vi "Spuler_interactive_lock_routine.vi"() -> ()   [LabVIEW 2012]
uses:
  <vilib>/DAQmx/write.llb/DAQmx Write (Digital 1D Bool NChan 1Samp 1Line).vi
  <vilib>/DAQmx/miscellaneous.llb/DAQmx Fill In Error Info.vi
  H2O_DIAL/LabVIEW-2012/Bristol WM V2_31b/CLDevIFace.dll
panel:
  out "On Diff read (nm)":dbl=2.73590208053065e-05 format="%_7g"
  in  "Lambda On Set (nm)":dbl=828.195 format="%#.5f"
  out "Online Lock":bool=TRUE
  out "Lambda On Read (nm)":dbl=828.1950273590209 format="%.5f"
  in  "Bristol In":i32=5
  in  "exit":bool
  out "WM Switch":bool=TRUE
  in  "WL Diff Allowed (nm)":dbl=5e-05 format="%#_15g"
  out "Off Diff read (nm)":dbl=2.4793750640128565e-05 format="%_7g"
  in  "Lambda Off Set (nm)":dbl=828.29425 format="%#.5f"
  out "Ofline Lock":bool=TRUE
  out "Lambda Off Read (nm)":dbl=828.2942747937507 format="%.5f"
  in  "Settings":T1={"Module"=enum."Etalon TEC", "OnLineTEC"=19.599694999999315, "OnLineLD"=0.15, "OffLineTEC"=17.258364999999106, "OffLineLD"=0.155, "EtalonTEC"=26.25, "TSOA-TEC"=18.0} {"OffLineLD" min=0.0 max=0.175 step=0.001 format="%.3p"; "OnLineLD" min=0.0 max=0.175 step=0.001 format="%.3p"; "TSOA-TEC" format="%.2g"; "EtalonTEC" format="%.2g"; "OffLineTEC" min=0.0 max=30.0 step=0.1 format="%.3g"; "OnLineTEC" min=0.0 max=30.0 step=0.1 format="%.3g"}
  out "Readings":T2={"OnLineTEC"=19.5938969, "OnLineLD"=0.150162116, "OffLineTEC"=17.2649479, "OffLineLD"=0.154738292, "EtalonTEC"=26.2012253, "TSOA-TEC"=18.0232182, "Pro8000"=TRUE, "OnLine TEC"=TRUE, "OnLine LD"=TRUE, "OffLine TEC"=TRUE, "OffLine LD"=TRUE, "Etalon TEC"=TRUE, "TSOA TEC"=TRUE} {"OffLineLD" format="%.4g"; "OnLineLD" format="%.4g"; "TSOA-TEC" format="%.3g"; "EtalonTEC" format="%.3g"; "OffLineTEC" format="%.3g"; "OnLineTEC" format="%.3g"}
  out "Bristol Out":i32=13
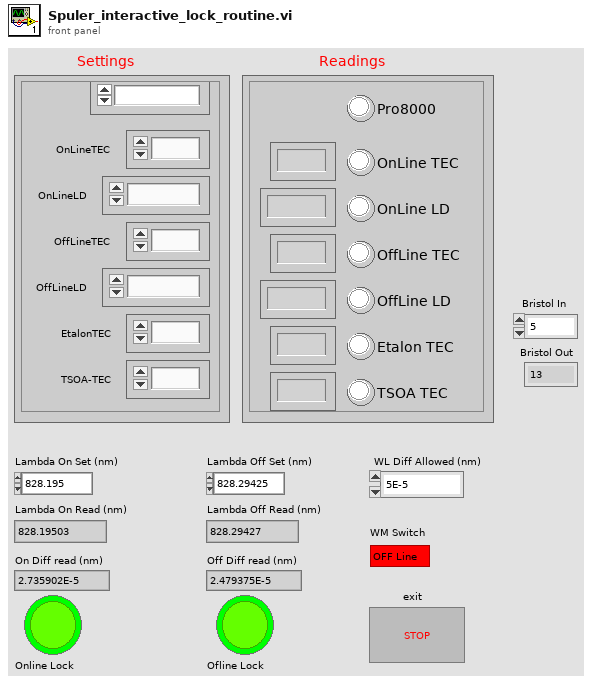
[diagram p1: front panel]
types:
  T1 = cluster{"Module":enum16{"On Line TEC", "On Line LD", "Off Line TEC", "Off Line LD", "Etalon TEC", "TSOA TEC"}, "OnLineTEC":dbl, "OnLineLD":dbl, "OffLineTEC":dbl, "OffLineLD":dbl, "EtalonTEC":dbl, "TSOA-TEC":dbl}
  T2 = cluster{"OnLineTEC":dbl, "OnLineLD":dbl, "OffLineTEC":dbl, "OffLineLD":dbl, "EtalonTEC":dbl, "TSOA-TEC":dbl, "Pro8000":bool, "OnLine TEC":bool, "OnLine LD":bool, "OffLine TEC":bool, "OffLine LD":bool, "Etalon TEC":bool, "TSOA TEC":bool}
  T3 = enum16{"Open_TL", "Close_TL", "Verify_ID", "TEC_Sensor", "SET", "READ", "ON", "OFF", "Set_Limits", "Read_Limits", "Enable_Status", "Read_Status"}
  T4 = enum16{"On Line TEC", "On Line LD", "Off Line TEC", "Off Line LD", "Etalon TEC", "TSOA TEC"}
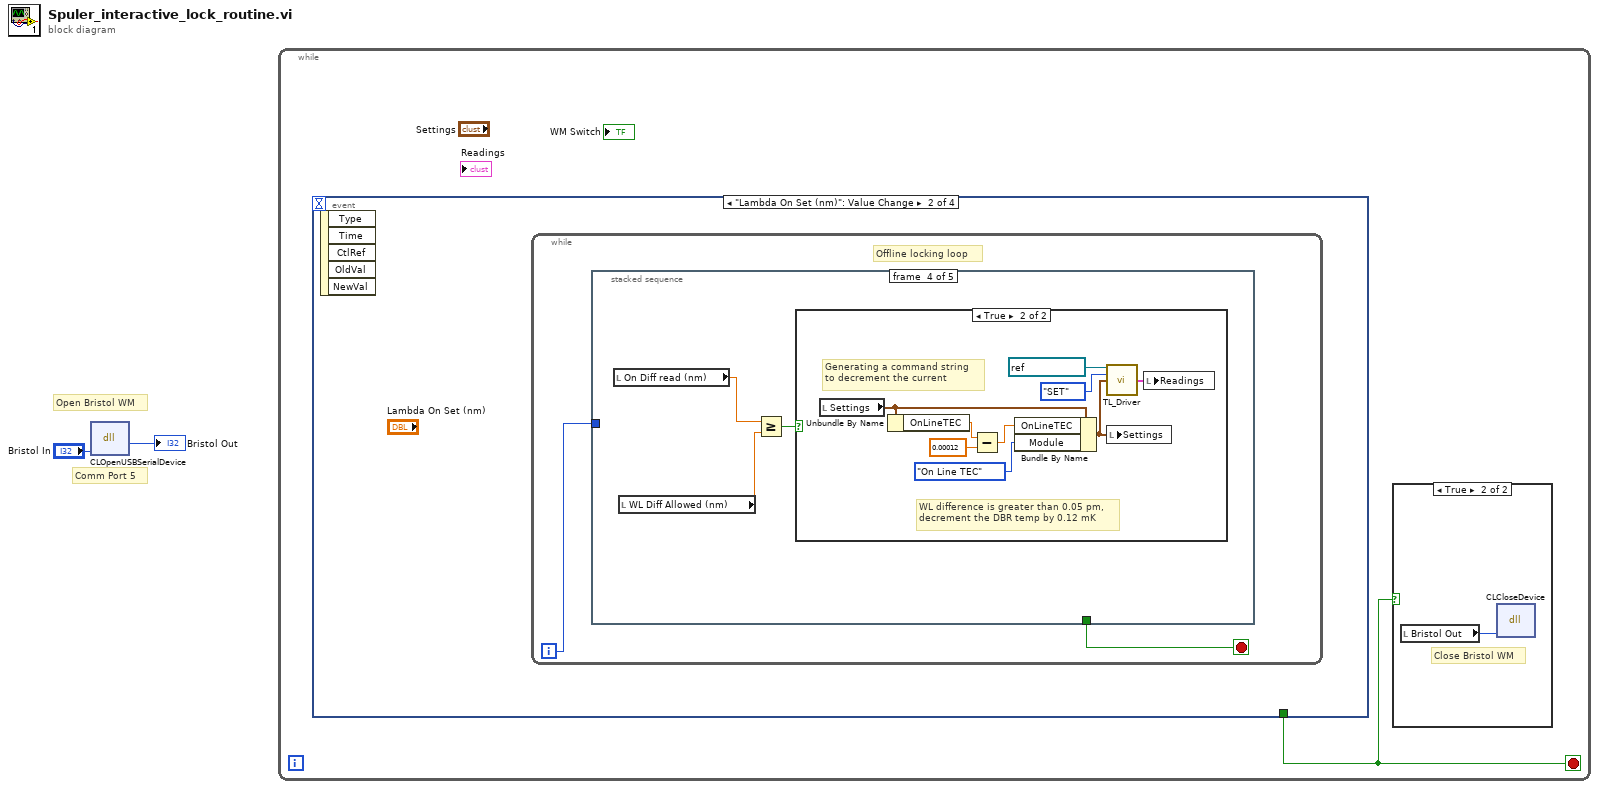
[diagram p0: block diagram]
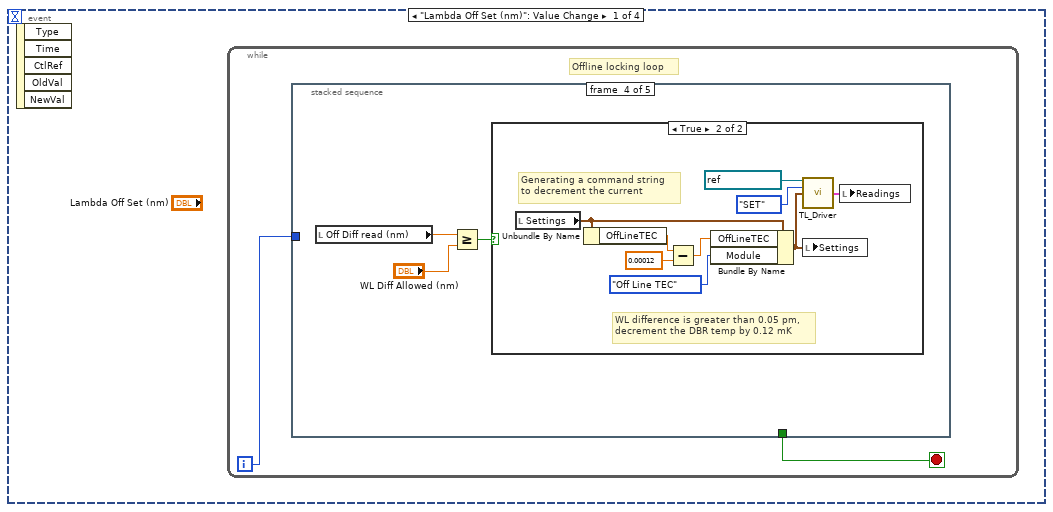
[diagram p3: hidden frame]
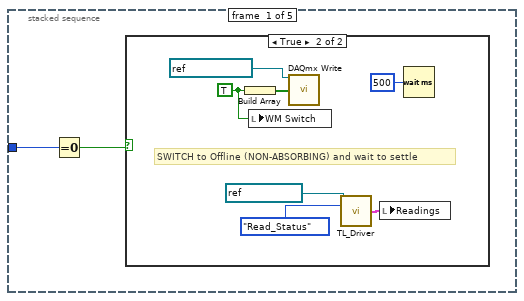
[diagram p4: hidden frame]
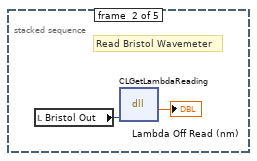
[diagram p6: hidden frame]
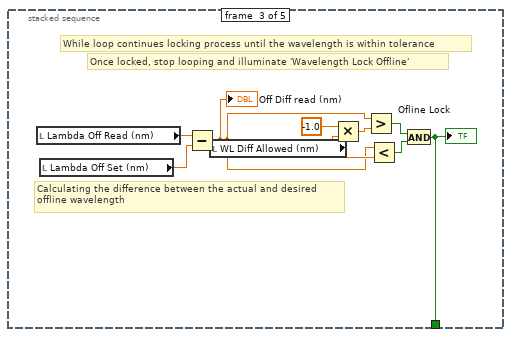
[diagram p7: hidden frame]
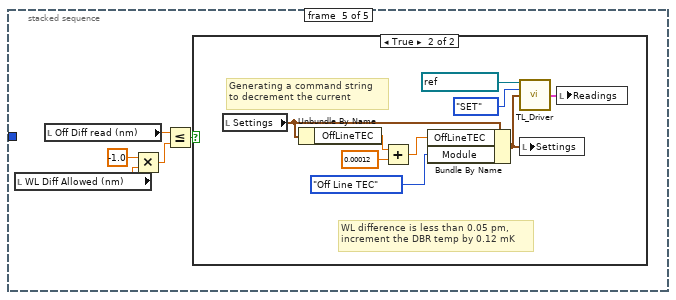
[diagram p9: hidden frame]
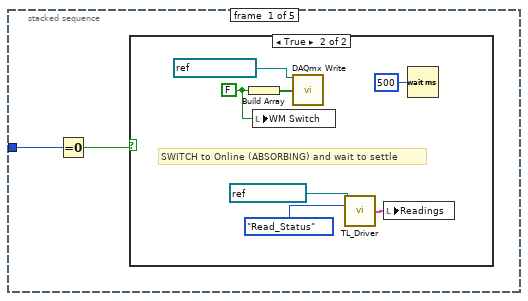
[diagram p11: hidden frame]
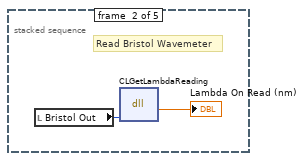
[diagram p13: hidden frame]
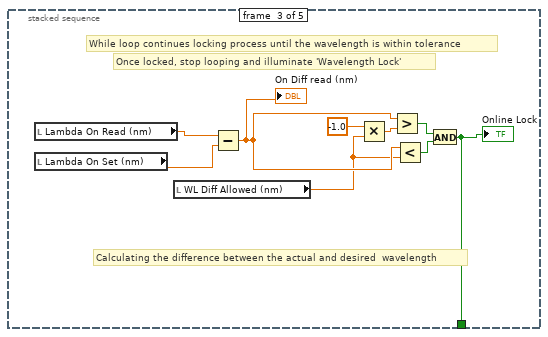
[diagram p14: hidden frame]
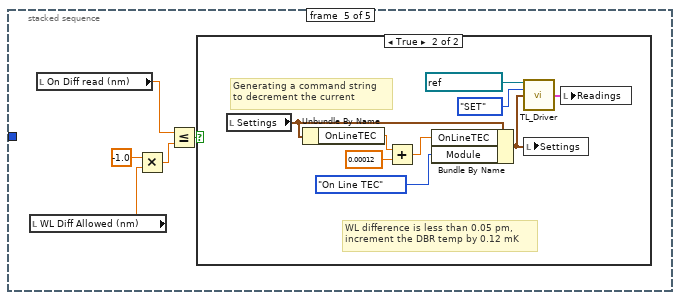
[diagram p16: hidden frame]
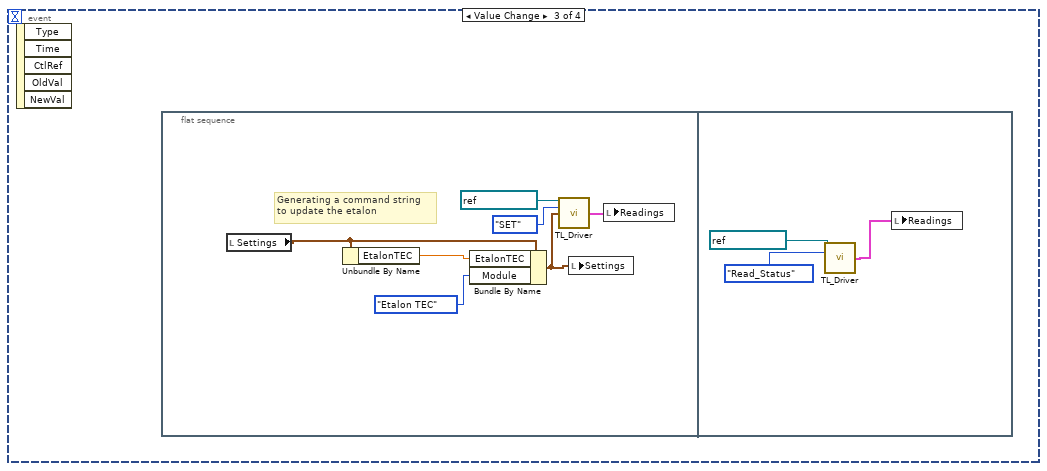
[diagram p18: hidden frame]
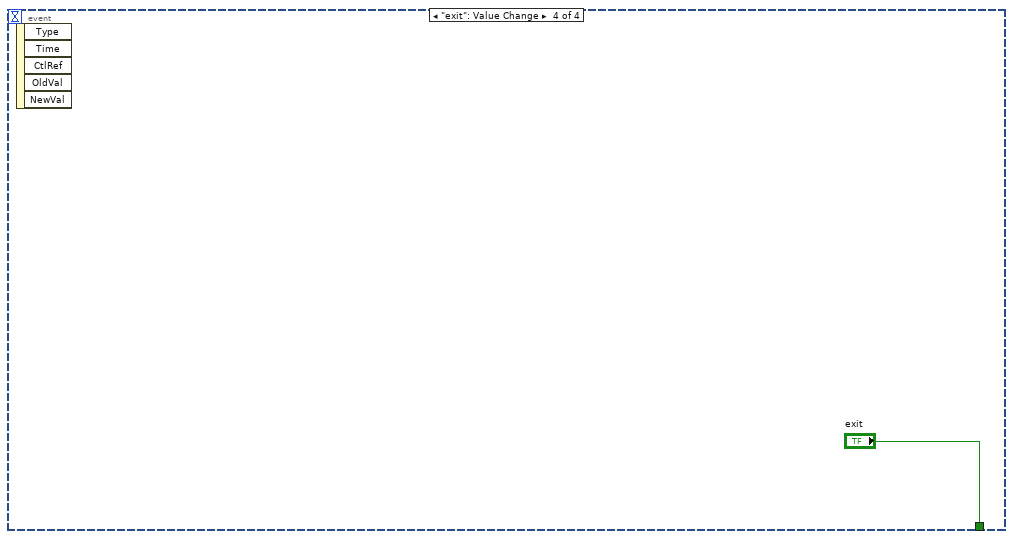
[diagram p19: hidden frame]
diagram:
  # "Comm Port 5"
  # "Open Bristol WM"
  n1 = dll-call lib="C:/H2O_DIAL/LabVIEW-2012/Bristol WM V2_31b/CLDevIface.dll" fn="CLOpenUSBSerialDevice"("commPort"="Bristol In") -> ("return type"=→"Bristol Out":i32)  [unwired: 4 in, 2 out]
  n2 = while {
    stop <- w3 stop-if-true
    n3 = event shown="[1] \"Lambda On Set (nm)\": Value Change" {
      selector: _ -> [_ _ _ _]
      dyn-events: _ -> [_ _ _ _]
      timeout: _ -> [_ _ _ _]
      tunnel: [_ _ _ "exit"] -> w3
      event "Lambda Off Set (nm)": Value Change {
        n4 = event-data() -> ()  [unwired: 1 in, 5 out]
        n5 = while {
          i -> [w5]
          stop <- w6 stop-if-true
          # "Offline locking loop"
          n6 = stacked-sequence {
            tunnel: [_ _ w20 _ _] -> w6
            tunnel: w5 -> [w8 _ _ _ _]
            frame #0 {
              n7 = Equal To 0?(x=w8) -> (x = 0?=w7:bool)
              n8 = case shown="True" w7 {
                frame False {
                }
                frame True {
                  w15 = TRUE ("Boolean")
                  # "SWITCH to Offline (NON-ABSORBING) and wait to settle"
                  n9 = Build Array(w15) -> (w10:bool[])
                  n10 = local write "WM Switch"(w15) -> ()
                  n11 = call-poly <vilib>:"DAQmx Write.vi"("task/channels in"=refnum<k21> "BristolWM", "data"=w10) -> ()  [unwired: 11 in, 3 out]
                  n12 = call "TL_Driver.vi"("Device In"=refnum<visa-resource-name> "ThorLabs", "Commands"=T3."Read_Status") -> ("Readings"=w12:T2)  [unwired: 10 in, 3 out]
                  n13 = local write "Readings"(w12) -> ()
                  n14 = Wait (ms)(milliseconds to wait=u32 500) -> ()  [unwired: 1 out]
                }
              }
            }
            frame #1 {
              # "Read Bristol Wavemeter"
              n15 = local read "Bristol Out"() -> (w16:i32)
              n16 = dll-call lib="C:/H2O_DIAL/LabVIEW-2012/Bristol WM V2_31b/CLDevIface.dll" fn="CLGetLambdaReading"("devHandle"=w16) -> ("return type"=→"Lambda Off Read (nm)":dbl)  [unwired: 4 in, 2 out]
            }
            frame #2 {
              # "Once locked, stop looping and illuminate 'Wavelength Lock Offline'"
              # "While loop continues locking process until the wavelength is within tolerance"
              # "Calculating the difference between the actual and desired \noffline wavelength"
              n17 = local read "Lambda Off Read (nm)"() -> (w18:dbl)
              n18 = local read "Lambda Off Set (nm)"() -> (w19:dbl)
              n19 = Subtract(x=w18, y=w19) -> (x-y=w21:dbl)
              "Off Diff read (nm)" <- w21
              n20 = local read "WL Diff Allowed (nm)"() -> (w25:dbl)
              n21 = Multiply(x=-1.0, y=w25) -> (x*y=w26:dbl)
              n22 = Greater?(x=w21, y=w26) -> (0:w22:bool)
              n23 = Less?(x=w21, y=w25) -> (x < y?=w23:bool)
              n24 = And(x=w22, y=w23) -> (x .and. y?=w20:bool)
              "Ofline Lock" <- w20
            }
            frame #3 {
              n25 = local read "Off Diff read (nm)"() -> (w29:dbl)
              n26 = Greater Or Equal?(x=w29, y="WL Diff Allowed (nm)") -> (x >= y?=w27:bool)
              n27 = case shown="True" w27 {
                frame False {
                  # "WL difference is not out of range, do nothing"
                }
                frame True {
                  # "Generating a command string\nto decrement the current"
                  # "WL difference is greater than 0.05 pm,\ndecrement the DBR temp by 0.12 mK"
                  n28 = local read "Settings"() -> (w34:T1)
                  n29 = Unbundle By Name(w34) -> ("OffLineTEC"=w35:dbl)
                  n30 = Subtract(x=w35, y=0.00012) -> (x-y=w36:dbl)
                  n31 = Bundle By Name(cluster=w34, "OffLineTEC"=w36, "Module"=T4."Off Line TEC") -> (w33:T1)
                  n32 = call "TL_Driver.vi"("Device In"=refnum<visa-resource-name> "ThorLabs", "Commands"=T3."SET", "Settings"=w33) -> ("Readings"=w30:T2)  [unwired: 9 in, 3 out]
                  n33 = local write "Settings"(w33) -> ()
                  n34 = local write "Readings"(w30) -> ()
                }
              }
            }
            frame #4 {
              n35 = local read "WL Diff Allowed (nm)"() -> (w40:dbl)
              n36 = local read "Off Diff read (nm)"() -> (w43:dbl)
              n37 = Multiply(x=-1.0, y=w40) -> (x*y=w39:dbl)
              n38 = Less Or Equal?(x=w43, y=w39) -> (x <= y?=w42:bool)
              n39 = case shown="True" w42 {
                frame False {
                  # "WL difference is not out of range, do nothing"
                }
                frame True {
                  # "Generating a command string\nto decrement the current"
                  # "WL difference is less than 0.05 pm,\nincrement the DBR temp by 0.12 mK"
                  n40 = local read "Settings"() -> (w47:T1)
                  n41 = Unbundle By Name(w47) -> ("OffLineTEC"=w49:dbl)
                  n42 = Add(x=w49, y=0.00012) -> (x+y=w50:dbl)
                  n43 = Bundle By Name(cluster=w47, "OffLineTEC"=w50, "Module"=T4."Off Line TEC") -> (w48:T1)
                  n44 = call "TL_Driver.vi"("Device In"=refnum<visa-resource-name> "ThorLabs", "Commands"=T3."SET", "Settings"=w48) -> ("Readings"=w44:T2)  [unwired: 9 in, 3 out]
                  n45 = local write "Settings"(w48) -> ()
                  n46 = local write "Readings"(w44) -> ()
                }
              }
            }
          }
        }
      }
      event "Lambda On Set (nm)": Value Change {
        n47 = event-data() -> ()  [unwired: 1 in, 5 out]
        n48 = while {
          i -> [w53]
          stop <- w54 stop-if-true
          # "Offline locking loop"
          n49 = stacked-sequence {
            tunnel: [_ _ w66 _ _] -> w54
            tunnel: w53 -> [w56 _ _ _ _]
            frame #0 {
              n50 = Equal To 0?(x=w56) -> (x = 0?=w55:bool)
              n51 = case shown="True" w55 {
                frame False {
                }
                frame True {
                  w63 = FALSE ("Boolean")
                  # "SWITCH to Online (ABSORBING) and wait to settle"
                  n52 = Build Array(w63) -> (w58:bool[])
                  n53 = local write "WM Switch"(w63) -> ()
                  n54 = call-poly <vilib>:"DAQmx Write.vi"("task/channels in"=refnum<k21> "BristolWM", "data"=w58) -> ()  [unwired: 11 in, 3 out]
                  n55 = call "TL_Driver.vi"("Device In"=refnum<visa-resource-name> "ThorLabs", "Commands"=T3."Read_Status") -> ("Readings"=w60:T2)  [unwired: 10 in, 3 out]
                  n56 = local write "Readings"(w60) -> ()
                  n57 = Wait (ms)(milliseconds to wait=u32 500) -> ()  [unwired: 1 out]
                }
              }
            }
            frame #1 {
              # "Read Bristol Wavemeter"
              n58 = local read "Bristol Out"() -> (w65:i32)
              n59 = dll-call lib="C:/H2O_DIAL/LabVIEW-2012/Bristol WM V2_31b/CLDevIface.dll" fn="CLGetLambdaReading"("devHandle"=w65) -> ("return type"=→"Lambda On Read (nm)":dbl)  [unwired: 4 in, 2 out]
            }
            frame #2 {
              # "Once locked, stop looping and illuminate 'Wavelength Lock'"
              # "While loop continues locking process until the wavelength is within tolerance"
              # "Calculating the difference between the actual and desired  wavelength"
              n60 = local read "Lambda On Read (nm)"() -> (w70:dbl)
              n61 = local read "Lambda On Set (nm)"() -> (w69:dbl)
              n62 = local read "WL Diff Allowed (nm)"() -> (w67:dbl)
              n63 = Subtract(x=w70, y=w69) -> (x-y=w68:dbl)
              "On Diff read (nm)" <- w68
              n64 = Multiply(x=-1.0, y=w67) -> (x*y=w74:dbl)
              n65 = Greater?(x=w68, y=w74) -> (0:w71:bool)
              n66 = Less?(x=w68, y=w67) -> (x < y?=w72:bool)
              n67 = And(x=w71, y=w72) -> (x .and. y?=w66:bool)
              "Online Lock" <- w66
            }
            frame #3 {
              n68 = local read "On Diff read (nm)"() -> (w75:dbl)
              n69 = local read "WL Diff Allowed (nm)"() -> (w76:dbl)
              n70 = Greater Or Equal?(x=w75, y=w76) -> (x >= y?=w77:bool)
              n71 = case shown="True" w77 {
                frame False {
                  # "WL difference is not out of range, do nothing"
                }
                frame True {
                  # "Generating a command string\nto decrement the current"
                  # "WL difference is greater than 0.05 pm,\ndecrement the DBR temp by 0.12 mK"
                  n72 = local read "Settings"() -> (w82:T1)
                  n73 = Unbundle By Name(w82) -> ("OnLineTEC"=w83:dbl)
                  n74 = Subtract(x=w83, y=0.00012) -> (x-y=w84:dbl)
                  n75 = Bundle By Name(cluster=w82, "OnLineTEC"=w84, "Module"=T4."On Line TEC") -> (w81:T1)
                  n76 = call "TL_Driver.vi"("Device In"=refnum<visa-resource-name> "ThorLabs", "Commands"=T3."SET", "Settings"=w81) -> ("Readings"=w78:T2)  [unwired: 9 in, 3 out]
                  n77 = local write "Settings"(w81) -> ()
                  n78 = local write "Readings"(w78) -> ()
                }
              }
            }
            frame #4 {
              n79 = local read "WL Diff Allowed (nm)"() -> (w87:dbl)
              n80 = local read "On Diff read (nm)"() -> (w88:dbl)
              n81 = Multiply(x=-1.0, y=w87) -> (x*y=w89:dbl)
              n82 = Less Or Equal?(x=w88, y=w89) -> (x <= y?=w91:bool)
              n83 = case shown="True" w91 {
                frame False {
                  # "WL difference is not out of range, do nothing"
                }
                frame True {
                  # "Generating a command string\nto decrement the current"
                  # "WL difference is less than 0.05 pm,\nincrement the DBR temp by 0.12 mK"
                  n84 = local read "Settings"() -> (w95:T1)
                  n85 = Unbundle By Name(w95) -> ("OnLineTEC"=w97:dbl)
                  n86 = Add(x=w97, y=0.00012) -> (x+y=w98:dbl)
                  n87 = Bundle By Name(cluster=w95, "OnLineTEC"=w98, "Module"=T4."On Line TEC") -> (w96:T1)
                  n88 = call "TL_Driver.vi"("Device In"=refnum<visa-resource-name> "ThorLabs", "Commands"=T3."SET", "Settings"=w96) -> ("Readings"=w92:T2)  [unwired: 9 in, 3 out]
                  n89 = local write "Settings"(w96) -> ()
                  n90 = local write "Readings"(w92) -> ()
                }
              }
            }
          }
        }
      }
      event "Settings.EtalonTEC": Value Change {
        n91 = event-data() -> ()  [unwired: 1 in, 5 out]
        n92 = flat-sequence {
          frame #0 {
            # "Generating a command string\nto update the etalon"
            n93 = local read "Settings"() -> (w104:T1)
            n94 = Unbundle By Name(w104) -> ("EtalonTEC"=w102:dbl)
            n95 = Bundle By Name(cluster=w104, "EtalonTEC"=w102, "Module"=T4."Etalon TEC") -> (w101:T1)
            n96 = call "TL_Driver.vi"("Device In"=refnum<visa-resource-name> "ThorLabs", "Commands"=T3."SET", "Settings"=w101) -> ("Readings"=w103:T2)  [unwired: 9 in, 3 out]
            n97 = local write "Settings"(w101) -> ()
            n98 = local write "Readings"(w103) -> ()
          }
          frame #1 {
            n99 = call "TL_Driver.vi"("Device In"=refnum<visa-resource-name> "ThorLabs", "Commands"=T3."Read_Status") -> ("Readings"=w110:T2)  [unwired: 10 in, 3 out]
            n100 = local write "Readings"(w110) -> ()
          }
        }
      }
      event "exit": Value Change {
        n101 = event-data() -> ()  [unwired: 1 in, 5 out]
      }
    }
    n102 = case shown="True" w3 {
      frame False {
      }
      frame True {
        # "Close Bristol WM"
        n103 = local read "Bristol Out"() -> (w4:i32)
        n104 = dll-call lib="C:/H2O_DIAL/LabVIEW-2012/Bristol WM V2_31b/CLDevIFace.dll" fn="CLCloseDevice"("CommPort"=w4) -> ()  [unwired: 5 in, 2 out]
      }
    }
  }
